vi "BallHolderControl.vi"   [LabVIEW 2015]
uses:
  <vilib>/Rock Robotics/WPI/Solenoid/WPI_SolenoidValue.ctl
  Utilities/MotorPositionGlobals.vi
  Utilities/GeneralGlobals.vi
  Utilities/VisionGlobals.vi
  <vilib>/Rock Robotics/WPI/Solenoid/WPI_SolenoidSetEnum.vi
types:
  T1 = typedef "WPI_SolenoidDevRef.ctl" = cluster{"DevStatus":errorcluster, "Pneumatics Control Module":u8, "Forward Solenoid Channel":T2, "Reverse Solenoid Channel":T2}
  T2 = typedef "WPI_SolenoidChannel.ctl" = enum8{"Solenoid 0", "Solenoid 1", "Solenoid 2", "Solenoid 3", "Solenoid 4", "Solenoid 5", "Solenoid 6", "Solenoid 7", "Invalid"}
  T3 = typedef "WPI_SolenoidValue.ctl" = enum16{"Off", "On", "Forward", "Reverse"}
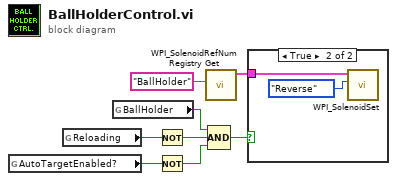
[diagram p0: block diagram]
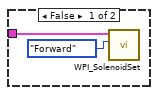
[diagram p2: hidden frame]
diagram:
  n1 = global read "VisionGlobals.vi" "AutoTargetEnabled?"() -> (w2:bool)
  n2 = global read "GeneralGlobals.vi" "Reloading"() -> (w6:bool)
  n3 = global read "MotorPositionGlobals.vi" "BallHolder"() -> (w5:bool)
  n4 = Not(x=w6) -> (.not. x?=w4:bool)
  n5 = Not(x=w2) -> (.not. x?=w1:bool)
  n6 = call <vilib>:"WPI_SolenoidRefNum Registry Get.vi"("refnum name"="BallHolder") -> ("SolenoidDevRef"=w7:T1)  [unwired: 9 in, 1 out]
  n7 = Compound Arithmetic op=AND(w5, w4, w1) -> (w3:bool)
  n8 = case shown="True" w3 {
    tunnel: w7 -> [w9 w11]
    frame False {
      n9 = call-poly <vilib>:"WPI_SolenoidSet.vi"("Value"=WPI_SolenoidValue."Forward", "SolenoidDevRef"=w9) -> ()  [unwired: 8 in, 2 out]
    }
    frame True {
      n10 = call-poly <vilib>:"WPI_SolenoidSet.vi"("Value"=WPI_SolenoidValue."Reverse", "SolenoidDevRef"=w11) -> ()  [unwired: 8 in, 2 out]
    }
  }
